vi "AnzeigeGV.vi"(0 "veränderte Methode benutzen":bool, 1 "Zykluslängen [s]":dbl[](array[numeric]), 2 "Cluster1":cluster{dbl[], dbl[], dbl[], dbl[]}, 3 "Big Ben, Methodenzeit, Zykluszeit0, Zykluszeit1, Zykluszeit2A, Zykluszeit2B":dbl[](array[numeric]), 4 "Zyklusnummern 0, 1, 2A, 2B":i32[](array[numeric]), 5 "Cluster2":cluster{dbl[], dbl[], dbl[], dbl[]}, 6 "AnzeigeEinstellungen":T1, 12 "dargestellte Größe 1":i32(ring)=1 items=["T-MainCol3", "T-Trap1", "T-Trap2", "T-Stirling", "T-PreCol1", "T-PreCol2", "T-MainCol1", "T-MainCol2", "T-T-Line2", "T-MI1", "T-MI2", "T-MI3", "T-MI4", "T-MI5", "T-MI6", "F-MFM1", "T-MainCol4", "T-BHorst1", "T-BHorst2", "T-BHorst3", "T-BHorst4", "T-Oven1", "T-Oven2", "T-T-Line1", "F-MFM2", "P-Me-HP", "P-Me-LP", "P-Vac", "Ref-Turbo", "I-MS-AC", "I-Trap1", "I-Trap2", "Mod2/AI0", "Mod2/AI1", "Mod2/AI2", "Mod2/AI3", "Mod2/AI4", "Mod2/AI5", "Mod2/AI6", "Mod2/AI7", "Mod2/AI8", "Mod2/AI9", "Mod2/AI10", "Mod2/AI11", "Mod2/AI12", "Mod2/AI13", "Mod2/AI14", "Mod2/AI15", "Mod2/AI16", "Mod2/AI17", "Mod2/AI18", "Mod2/AI19", "Mod2/AI20", "Mod2/AI21", "Mod2/AI22", "Mod2/AI23", "Mod2/AI24", "Mod2/AI25", "Mod2/AI26", "Mod2/AI27", "Mod2/AI28", "Mod2/AI29", "Mod2/AI30", "Mod2/AI31", "Mod3/AI0", "Mod3/AI1", "Mod3/AI2", "Mod3/AI3", "Mod3/AI4", "Mod3/AI5", "Mod3/AI6", "Mod3/AI7", "Mod3/AI8", "Mod3/AI9", "Mod3/AI10", "Mod3/AI11", "Mod3/AI12", "Mod3/AI13", "Mod3/AI14", "Mod3/AI15", "Mod3/AI16", "Mod3/AI17", "Mod3/AI18", "Mod3/AI19", "Mod3/AI20", "Mod3/AI21", "Mod3/AI22", "Mod3/AI23", "Mod3/AI24", "Mod3/AI25", "Mod3/AI26", "Mod3/AI27", "Mod3/AI28", "Mod3/AI29", "Mod3/AI30", "Mod3/AI31", "U_Widr.Trap1 [V]", "Temp.Trap1 [°C]", "U_Widr.Trap2 [V]", "Temp.Trap2 [°C]", "Temp.Mach1 [°C]", "Temp.Mach2 [°C]", "MFC1B", "PressContr1A", "PressContr1B", "PressContr1C", "MFC1A", "PressContr1D", "MFC1A Integriert"], 14 "Zeitachse1":i32(ring)=1 items=["Zykluszeit [s] Mod0", "Zykluszeit [s] Mod1", "Zykluszeit [s] Mod2A", "Zykluszeit [s] Mod2B"], 16 "dargestellte Größe 2":i32(ring)=1 items=["T-MainCol3", "T-Trap1", "T-Trap2", "T-Stirling", "T-PreCol1", "T-PreCol2", "T-MainCol1", "T-MainCol2", "T-T-Line2", "T-MI1", "T-MI2", "T-MI3", "T-MI4", "T-MI5", "T-MI6", "F-MFM1", "T-MainCol4", "T-BHorst1", "T-BHorst2", "T-BHorst3", "T-BHorst4", "T-Oven1", "T-Oven2", "T-T-Line1", "F-MFM2", "P-Me-HP", "P-Me-LP", "P-Vac", "Ref-Turbo", "I-MS-AC", "I-Trap1", "I-Trap2", "Mod2/AI0", "Mod2/AI1", "Mod2/AI2", "Mod2/AI3", "Mod2/AI4", "Mod2/AI5", "Mod2/AI6", "Mod2/AI7", "Mod2/AI8", "Mod2/AI9", "Mod2/AI10", "Mod2/AI11", "Mod2/AI12", "Mod2/AI13", "Mod2/AI14", "Mod2/AI15", "Mod2/AI16", "Mod2/AI17", "Mod2/AI18", "Mod2/AI19", "Mod2/AI20", "Mod2/AI21", "Mod2/AI22", "Mod2/AI23", "Mod2/AI24", "Mod2/AI25", "Mod2/AI26", "Mod2/AI27", "Mod2/AI28", "Mod2/AI29", "Mod2/AI30", "Mod2/AI31", "Mod3/AI0", "Mod3/AI1", "Mod3/AI2", "Mod3/AI3", "Mod3/AI4", "Mod3/AI5", "Mod3/AI6", "Mod3/AI7", "Mod3/AI8", "Mod3/AI9", "Mod3/AI10", "Mod3/AI11", "Mod3/AI12", "Mod3/AI13", "Mod3/AI14", "Mod3/AI15", "Mod3/AI16", "Mod3/AI17", "Mod3/AI18", "Mod3/AI19", "Mod3/AI20", "Mod3/AI21", "Mod3/AI22", "Mod3/AI23", "Mod3/AI24", "Mod3/AI25", "Mod3/AI26", "Mod3/AI27", "Mod3/AI28", "Mod3/AI29", "Mod3/AI30", "Mod3/AI31", "U_Widr.Trap1 [V]", "Temp.Trap1 [°C]", "U_Widr.Trap2 [V]", "Temp.Trap2 [°C]", "Temp.Mach1 [°C]", "Temp.Mach2 [°C]", "MFC1B", "PressContr1A", "PressContr1B", "PressContr1C", "MFC1A", "PressContr1D", "MFC1A Integriert"], 18 "Zeitachse2":i32(ring)=1 items=["Zykluszeit [s] Mod0", "Zykluszeit [s] Mod1", "Zykluszeit [s] Mod2A", "Zykluszeit [s] Mod2B"]) -> (19 "Anzeige2":cluster{dbl[], dbl[]}(graph), 20 "Cluster1":cluster{dbl[], dbl[], dbl[], dbl[]}, 21 "x1Inkr":dbl, 22 "Cluster2":cluster{dbl[], dbl[], dbl[], dbl[]}, 23 "Anzeige1":cluster{dbl[], dbl[]}(graph), 24 "AnzeigeEinstellungen":T1, 25 "x2Max":dbl, 26 "x2Inkr":dbl, 27 "x1Max":dbl)   [LabVIEW 2017]
uses:
  GVMWHorst.vi
  GVMethodenwechsel.vi
  GVHK1Hz.vi
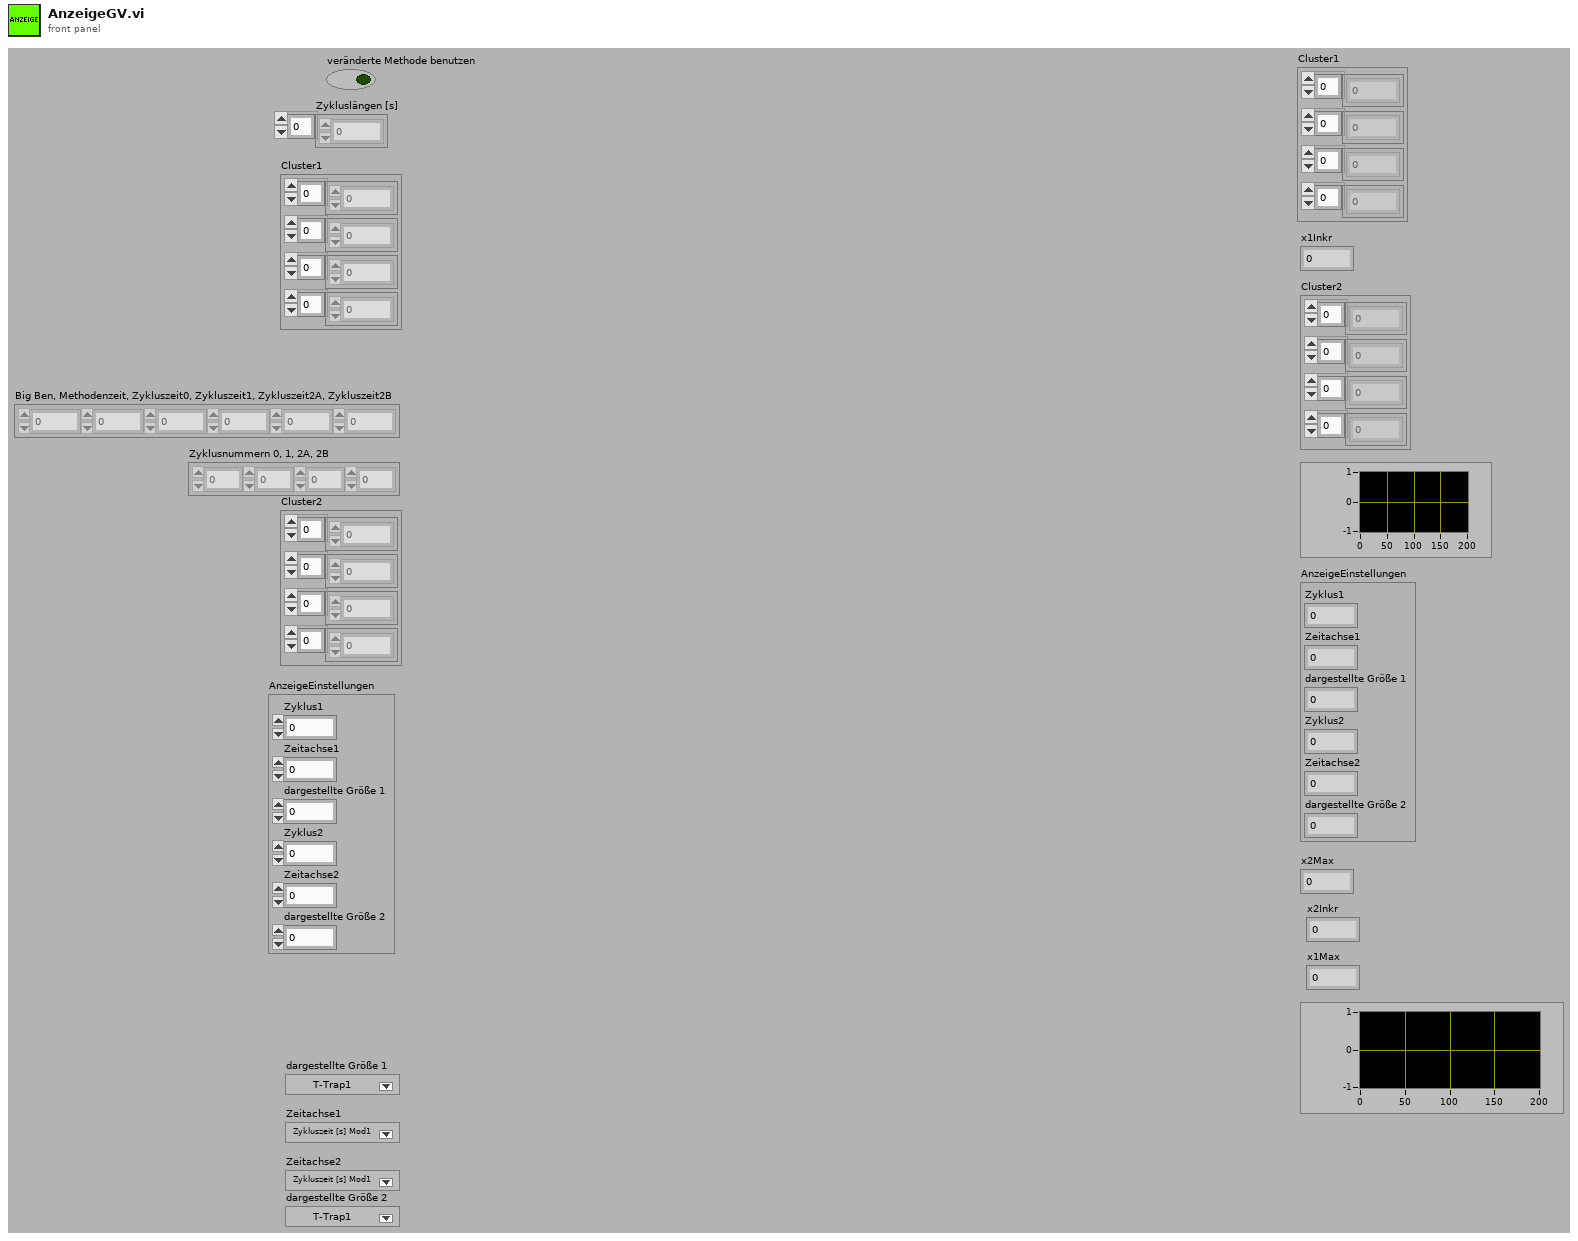
[diagram p1: front panel]
types:
  T1 = cluster{"Zyklus1":i32, "Zeitachse1":i32, "dargestellte Größe 1":i32, "Zyklus2":i32, "Zeitachse2":i32, "dargestellte Größe 2":i32}
  T2 = cluster{i32, "Zeitachse1":i32, "dargestellte Größe 1":i32, i32, "Zeitachse2":i32, "dargestellte Größe 2":i32}
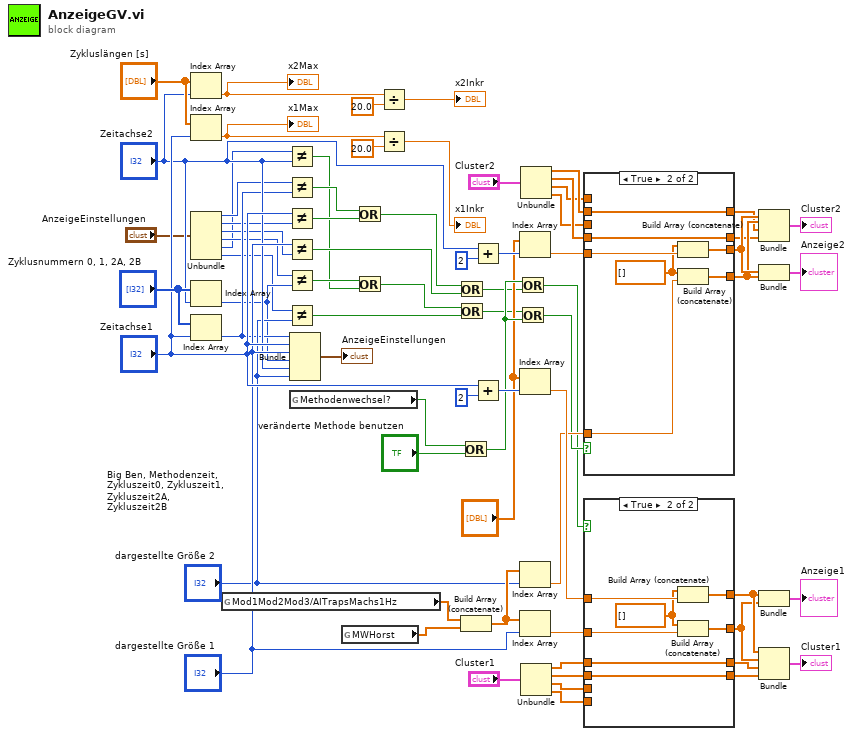
[diagram p0: block diagram]
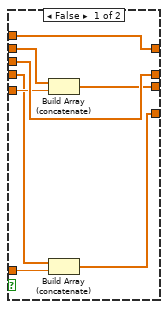
[diagram p2: hidden frame]
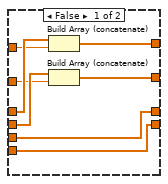
[diagram p3: hidden frame]
diagram:
  n1 = Index Array(array="Zykluslängen [s]", index="Zeitachse2") -> (element=w24:dbl)
  "x2Max" <- w24
  n2 = Index Array(array="Zykluslängen [s]", index="Zeitachse1") -> (element=w22:dbl)
  "x1Max" <- w22
  n3 = Unbundle("AnzeigeEinstellungen") -> ("Zyklus1"=w14:i32, "Zeitachse1"=w12:i32, "dargestellte Größe 1"=w11:i32, "Zyklus2"=w10:i32, "Zeitachse2"=w8:i32, "dargestellte Größe 2"=w7:i32)
  n4 = Index Array(array="Zyklusnummern 0, 1, 2A, 2B", index="Zeitachse2") -> (element=w9:i32)
  n5 = Index Array(array="Zyklusnummern 0, 1, 2A, 2B", index="Zeitachse1") -> (element=w13:i32)
  n6 = global read "GVHK1Hz.vi" "Mod1Mod2Mod3/AITrapsMachs1Hz"() -> (w1:dbl[])
  n7 = Not Equal?(x=w8, y="Zeitachse2") -> (x != y?=w59:bool)
  n8 = Not Equal?(x=w14, y=w13) -> (x != y?=w68:bool)
  n9 = Not Equal?(x="Zeitachse1", y=w12) -> (x != y?=w66:bool)
  n10 = Not Equal?(x="dargestellte Größe 1", y=w11) -> (x != y?=w65:bool)
  n11 = Not Equal?(x=w10, y=w9) -> (x != y?=w60:bool)
  n12 = Not Equal?(x=w7, y="dargestellte Größe 2") -> (x != y?=w57:bool)
  n13 = Bundle(w13, "Zeitachse1"="Zeitachse1", "dargestellte Größe 1"="dargestellte Größe 1", w9, "Zeitachse2"="Zeitachse2", "dargestellte Größe 2"="dargestellte Größe 2") -> (→"AnzeigeEinstellungen":T2)  [unwired: 1 in]
  n14 = global read "GVMethodenwechsel.vi" "Methodenwechsel?"() -> (w4:bool)
  n15 = global read "GVMWHorst.vi" "MWHorst"() -> (w5:dbl[])
  n16 = Or(x=w68, y=w66) -> (x .or. y?=w67:bool)
  n17 = Or(x=w60, y=w59) -> (x .or. y?=w58:bool)
  n18 = Divide(x=w24, y=20.0) -> (x/y=→"x2Inkr":dbl)
  n19 = Divide(x=w22, y=20.0) -> (x/y=→"x1Inkr":dbl)
  n20 = Or(x=w67, y=w65) -> (x .or. y?=w3:bool)
  n21 = Or(x=w58, y=w57) -> (x .or. y?=w2:bool)
  n22 = Or(x=w4, y="veränderte Methode benutzen") -> (x .or. y?=w49:bool)
  n23 = Build Array (concatenate)(w1, w5) -> (w63:dbl[])
  n24 = Add(x="Zeitachse2", y=2) -> (x+y=w54:i32)
  n25 = Add(x="Zeitachse1", y=2) -> (x+y=w53:i32)
  n26 = Or(x=w49, y=w3) -> (x .or. y?=w48:bool)
  n27 = Or(x=w2, y=w49) -> (x .or. y?=w50:bool)
  n28 = Index Array(array="Big Ben, Methodenzeit, Zykluszeit0, Zykluszeit1, Zykluszeit2A, Zykluszeit2B", index=w54) -> (element=w61:dbl)
  n29 = Index Array(array="Big Ben, Methodenzeit, Zykluszeit0, Zykluszeit1, Zykluszeit2A, Zykluszeit2B", index=w53) -> (element=w70:dbl)
  n30 = Index Array(array=w63, index="dargestellte Größe 2") -> (element=w62:dbl)
  n31 = Index Array(array=w63, index="dargestellte Größe 1") -> (element=w69:dbl)
  n32 = Unbundle("Cluster2") -> (w47:dbl[], w46:dbl[], w45:dbl[], w44:dbl[])
  n33 = Unbundle("Cluster1") -> (w38:dbl[], w37:dbl[], w36:dbl[], w35:dbl[])
  n34 = case shown="True" w50 {
    tunnel: w47 -> [w77 w81]
    tunnel: [w75 w85] -> w43
    tunnel: [w72 w82] -> w42
    tunnel: w45 -> [w79 _]
    tunnel: [w79 w81] -> w41
    tunnel: w44 -> [w78 _]
    tunnel: [w78 w80] -> w40
    tunnel: w61 -> [w76 w86]
    tunnel: w46 -> [w74 w80]
    tunnel: w62 -> [w73 w83]
    frame False {
      n35 = Build Array (concatenate)(w77, w76) -> (w75:dbl[])
      n36 = Build Array (concatenate)(w74, w73) -> (w72:dbl[])
    }
    frame True {
      w84 = dbl[] []
      n37 = Build Array (concatenate)(w84, w86) -> (w85:dbl[])
      n38 = Build Array (concatenate)(w84, w83) -> (w82:dbl[])
    }
  }
  n39 = case shown="True" w48 {
    tunnel: w38 -> [w92 w96]
    tunnel: [w90 w100] -> w34
    tunnel: [w87 w97] -> w33
    tunnel: w36 -> [w94 _]
    tunnel: [w94 w96] -> w32
    tunnel: w35 -> [w93 _]
    tunnel: [w93 w95] -> w31
    tunnel: w70 -> [w91 w101]
    tunnel: w37 -> [w89 w95]
    tunnel: w69 -> [w88 w98]
    frame False {
      n40 = Build Array (concatenate)(w92, w91) -> (w90:dbl[])
      n41 = Build Array (concatenate)(w89, w88) -> (w87:dbl[])
    }
    frame True {
      w99 = dbl[] []
      n42 = Build Array (concatenate)(w99, w101) -> (w100:dbl[])
      n43 = Build Array (concatenate)(w99, w98) -> (w97:dbl[])
    }
  }
  n44 = Bundle(w43, w42, w41, w40) -> (→"Cluster2":cluster{dbl[], dbl[], dbl[], dbl[]})  [unwired: 1 in]
  n45 = Bundle(w43, w42) -> (→"Anzeige2":cluster{dbl[], dbl[]})  [unwired: 1 in]
  n46 = Bundle(w34, w33) -> (→"Anzeige1":cluster{dbl[], dbl[]})  [unwired: 1 in]
  n47 = Bundle(w34, w33, w32, w31) -> (→"Cluster1":cluster{dbl[], dbl[], dbl[], dbl[]})  [unwired: 1 in]
